vi "Rerun Tests.vi"(8 "error in (no error)":errorcluster, 11 "Storage":refnum<class "Test Event Storage.lvclass">) -> (0 "error out":errorcluster, 2 "Called Run Tests in Active Project":bool)   [LabVIEW 2020, in "Caraya.lvlib" / "Basic Test Manager.lvclass"]
uses:
  Basic Test Manager.lvclass
  Test Event Storage/Test Event Storage.lvclass
  subVIs/Run Tests (Project).vi
  <vilib>/regexp/Match Regular Expression.xnode
  Caraya.lvlib
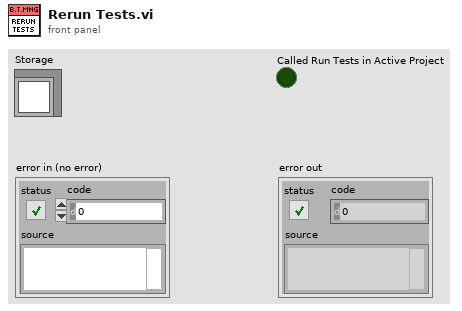
[diagram p1: front panel]
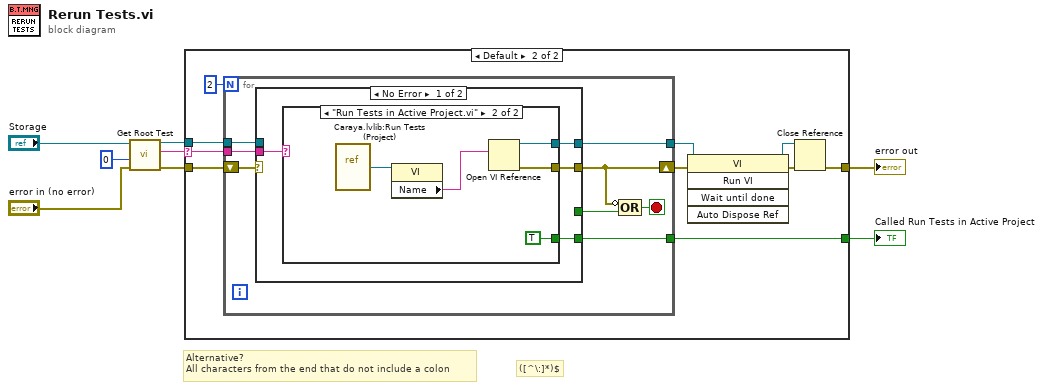
[diagram p0: block diagram]
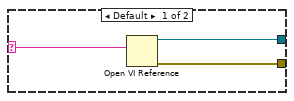
[diagram p3: hidden frame]
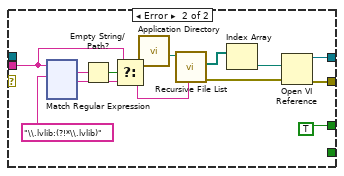
[diagram p4: hidden frame]
diagram:
  # "([^\\:]*)$"
  # "Alternative?\nAll characters from the end that do not include a colon"
  n1 = call-dynamic "Get Root Test.vi"("error in (no error)"="error in (no error)", "index (0: root)"=0, "Test Event Storage in"="Storage") -> ("error out"=w8:errorcluster, "Test"=w2:string, "Test Event Storage out"=w6:refnum<class "Test Event Storage.lvclass">)  [unwired: 6 in]
  n2 = case shown="Default" w2 {
    selector: w2 -> [_ w11]
    tunnel: w8 -> [w9 w14]
    tunnel: w6 -> [_ w13]
    tunnel: [w9 w12] -> w3
    tunnel: [_ w10] -> w1
    frame "" {
    }
    frame Default {
      n3 = for {
        N: 2 -> [_]
        tunnel: [w26] -> w15
        tunnel: w11 -> [w25]
        tunnel: w13 -> [w24]
        shift-right: [w21] -> w17
        shift-left: w14 -> [w27]
        tunnel: [w20] -> w10
        stop <- w22 stop-if-true
        n4 = case shown="No Error" w27 {
          tunnel: [w31 w52] -> w21
          tunnel: [w30 w51] -> w26
          tunnel: w25 -> [w29 w46]
          tunnel: w24 -> [_ _]
          tunnel: [_ TRUE] -> w23
          tunnel: [w28 _] -> w20
          frame No Error {
            n5 = case shown="\"Run Tests in Active Project.vi\"" w29 {
              selector: w29 -> [w32 _]
              tunnel: [w34 w38] -> w31
              tunnel: [w33 w39] -> w30
              tunnel: [_ TRUE] -> w28
              frame Default {
                n6 = Open VI Reference(vi path=w32) -> (vi reference=w33:refnum<vi>, error out=w34:errorcluster)  [unwired: 5 in]
              }
              frame "Run Tests in Active Project.vi" {
                n7 = vi-ref "Caraya.lvlib:Run Tests (Project).vi"() -> (w37:refnum<vi>)
                n8 = property class="VI"(reference=w37) -> ("Name"=w36:string)  [unwired: 1 in, 2 out]
                n9 = Open VI Reference(vi path=w36) -> (vi reference=w39:refnum<vi>, error out=w38:errorcluster)  [unwired: 5 in]
              }
            }
          }
          frame Error {
            n10 = xnode "Match Regular Expression"("input string"=w46, "regular expression"="\\.lvlib:(?!*\\.lvlib)") -> ("whole match"=w49:string, "after match"=w47:string)  [unwired: 4 in, 3 out]
            n11 = Empty String/Path?(string/path=w49) -> (empty?=w48:bool)
            n12 = Select(t=w46, s=w48, f=w47) -> (s? t:f=w44:string)
            n13 = call <vilib>:"Application Directory.vi"() -> ("Application Directory"=w45:path)
            n14 = call <vilib>:"Recursive File List.vi"("pattern"=w44, "Folder Path"=w45) -> ("error out"=w42:errorcluster, "All Files in Dir"=w41:path[])  [unwired: 5 in, 3 out]
            n15 = Index Array(array=w41) -> (element=w43:path)  [unwired: 1 in]
            n16 = Open VI Reference(vi path=w43, error in (no error)=w42) -> (vi reference=w51:refnum<vi>, error out=w52:errorcluster)  [unwired: 4 in]
          }
        }
        n17 = Compound Arithmetic op=OR(invert w21, w23) -> (w22:bool)
      }
      n18 = invoke class="VI" method="Run VI"(reference=w15, error in=w17) -> (reference out=w16:refnum<vi>, error out=w18:errorcluster)  [unwired: 3 in, 3 out]
      n19 = Close Reference(reference=w16, error in (no error)=w18) -> (error out=w12:errorcluster)
    }
  }
  "error out" <- w3
  "Called Run Tests in Active Project" <- w1
